vi "time-stringSD.vi"() -> (0 "time":string)   [LabVIEW 2015]
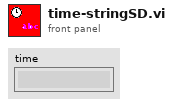
[diagram p1: front panel]
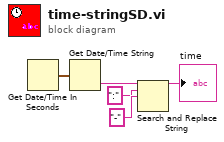
[diagram p0: block diagram]
diagram:
  n1 = Get Date/Time In Seconds() -> (seconds since 1Jan1904=w4:timestamp)
  n2 = Get Date/Time String(seconds (now)=w4) -> (time string=w5:string)  [unwired: 2 in, 1 out]
  n3 = Search and Replace String(input string=w5, search string=":", replace string="-" ("replace string (\"\")")) -> (result string=→"time":string)  [unwired: 5 in, 3 out]
